vi "TDT-Close ActiveX.vi"(11 "error in (no error)":errorcluster) -> (15 "error out":errorcluster)   [LabVIEW 2020]
uses:
  TDT-Globals.vi
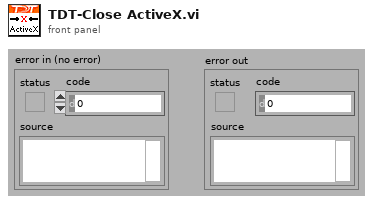
[diagram p1: front panel]
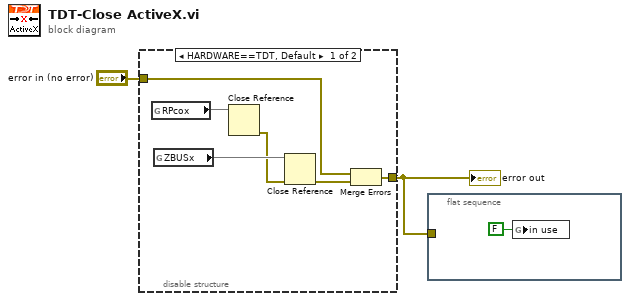
[diagram p0: block diagram]
diagram:
  n1 = disable-structure shown="HARDWARE==TDT, Default" {
    disable-tunnel: "error in (no error)" -> [w5 w9]
    disable-tunnel: [w3 w9] -> w1
    frame condition #0 (active) {
      n2 = global read "TDT-Globals.vi" "RPcox"() -> (w8)
      n3 = global read "TDT-Globals.vi" "ZBUSx"() -> (w7)
      n4 = Close Reference(reference=w8) -> (error out=w6:errorcluster)  [unwired: 1 in]
      n5 = Close Reference(reference=w7, error in (no error)=w6) -> (error out=w4:errorcluster)
      n6 = Merge Errors(w5, w4) -> (w3:errorcluster)
    }
    frame condition #1 {
    }
  }
  "error out" <- w1
  n7 = flat-sequence {
    tunnel: w1 -> [_]
    frame #0 {
      n8 = global write "TDT-Globals.vi" "in use"(FALSE ("in use")) -> ()
    }
  }
